vi "GetContolRefByLabel(FromVIRef).vi"(8 "error in (no error)":errorcluster, 10 "CntrlLabel":string, 11 "VI in":refnum<vi>) -> (0 "error out":errorcluster, 2 "Found?":bool, 3 "Control out":refnum<vi>)   [LabVIEW 2013]
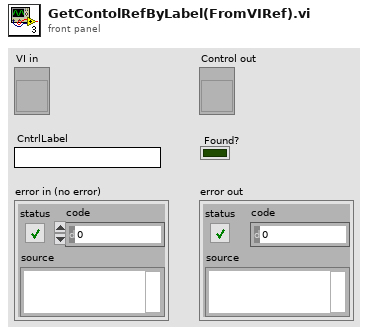
[diagram p1: front panel]
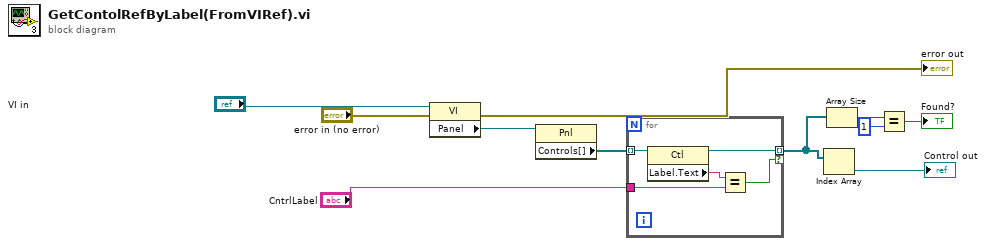
[diagram p0: block diagram]
diagram:
  n1 = property class="VI"(reference="VI in", error in="error in (no error)") -> (error out=→"error out":errorcluster, "Panel"=w2:refnum<vi>)  [unwired: 1 out]
  n2 = property class="Pnl"(reference=w2) -> ("Controls[]"=w3:refnum<vi>[])  [unwired: 1 in, 2 out]
  n3 = for {
    tunnel: w3 -> [w16] mode=indexing
    tunnel: [w14] -> w4 mode=indexing if=w13
    tunnel: "CntrlLabel" -> [w12]
    n4 = property class="Ctl"(reference=w16) -> (reference out=w14:refnum<vi>, "Label.Text"=w15:string)  [unwired: 1 in, 1 out]
    n5 = Equal?(x=w15, y=w12) -> (x = y?=w13:bool)
  }
  n6 = Index Array(array=w4) -> (element=→"Control out":refnum<vi>)  [unwired: 1 in]
  n7 = Array Size(array=w4) -> (size(s)=w5:i32)
  n8 = Equal?(x=w5, y=1) -> (x = y?=→"Found?":bool)
